vi "sv_Peak View Amplitude (Array).vi"(7 "peak units":enum16{"EU rms", "EU peak", "EU peak-peak"}(ring), 8 "error in (no error)":errorcluster, 9 "spectrum info":T1={"channel name"="", "description"="", "x-axis units"=0, "spectral info"={"spectrum type"=enum."Power [Magnitude^2]", "linear/dB"=enum."linear", "window"=0, "window size"=0, "FFT size"=0}, "engineering units"=0, "custom label"="", "dB reference [EU]"=0.0, "peak units"=enum."rms", "weighting filter"=0, "spectral density?"=FALSE, "unit label"="", "spectrum skewed?"=FALSE, "complimentary spectrum units"=enum."none"} {"x-axis units" items=["Time (s)"=0, "Frequency-CB (Hz)"=1, "Frequency-CPB (Hz)"=1248, "Frequency-Arbitrary (Hz)"=2357, "Quefrency (s)"=2, "Revolutions (rev)"=3, "Order"=4, "Speed (RPM)"=11, "Speed (rad/s)"=21, "Index"=65535]; "weighting filter" items=["Linear", "A-weighting", "B-weighting", "C-weighting", "ITU-R 468-4", "Dolby", "CCITT", "C-message", "Wb", "Wc", "Wd", "We", "Wf", "Wh", "Wj", "Wk", "Wm", "AES17 20 kHz lowpass", "AES17 40 kHz lowpass", "AES17 20 kHz highpass", "AES17 40 kHz highpass"]; "dB reference [EU]" format="%.2f"; "engineering units" items=["custom..."=0, "V"=1, "A"=21, "C"=30, "pC"=31, "s"=32, "-"=29, "Pa"=2, "N"=20, "g"=3, "m/s^2"=4, "m/s"=5, "m"=6, "mm/s"=12, "mm"=13, "micron/s"=14, "micron"=15, "in/s^2"=7, "in/s"=8, "in"=9, "mil/s"=10, "mil"=11, "rad/s^2"=16, "rad/s"=17, "rad"=18, "deg/s^2"=26, "deg/s"=27, "deg"=28, "RPM"=22, "cycle/s^2"=23, "Hz"=24, "cycle"=25, "strain"=19]; "spectral info"."window" items=["None "=0, "Hanning"=1, "Hamming"=2, "Blackman-Harris"=3, "Exact Blackman"=4, "Blackman"=5, "Flat Top"=6, "4 Term B-Harris "=7, "7 Term B-Harris"=8, "Low Sidelobe"=9, "Force - Exponential"=10, "Gaussian"=62]}, 11 "peak amplitudes [EU pk]":dbl[](array[numeric]) format="%.2f") -> (0 "error out":errorcluster, 3 "converted peak amplitudes":dbl[](array[numeric]) format="%.2f", 5 "unit label":string)   [LabVIEW 2017, in "SoundVib_Distortion.lvlib"]
uses:
  <vilib>/addons/Sound and Vibration/svt_Distortion/SoundVib_Distortion.lvlib
  <vilib>/addons/_NISVFA/_Shared subVIs/Controls/svc_Spectrum Info.ctl
  <vilib>/addons/_NISVFA/_Shared subVIs/Controls/svc_X-Axis Units.ctl
  <vilib>/addons/_NISVFA/_Shared subVIs/Controls/svc_Spectrum Type.ctl
  <vilib>/addons/_NISVFA/_Shared subVIs/Controls/svc_Engineering Units Text Ring.ctl
  <vilib>/addons/_NISVFA/_Shared subVIs/Controls/svc_Weighting Filter Text Ring.ctl
  <vilib>/addons/_NISVFA/_Shared subVIs/Controls/svc_Complimentary Spectrum Units.ctl
  <vilib>/addons/_NISVFA/_Shared subVIs/Common/svc_Get Weighting Enum and Labels.vi
  <vilib>/addons/_NISVFA/_Shared subVIs/Common/svc_Unit Label Lexical Class.vi
  <vilib>/addons/_NISVFA/_Shared subVIs/Common/svc_Engineering Units to Unit Label.vi
  <vilib>/addons/_NISVFA/_Shared subVIs/Common/svc_Format Value (DBL).vi
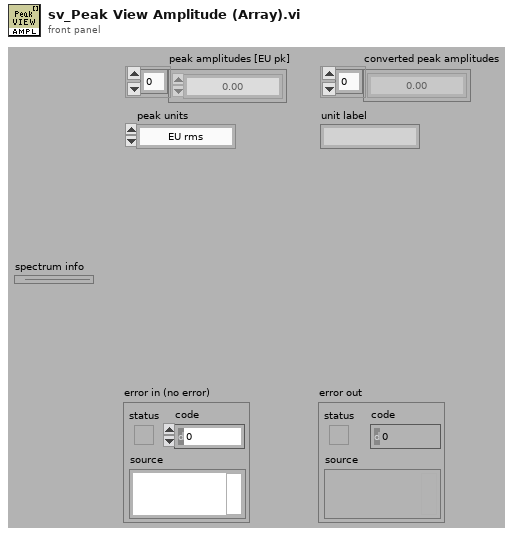
[diagram p1: front panel]
types:
  T1 = typedef "svc_Spectrum Info.ctl" = cluster{"channel name":string, "description":string, "x-axis units":T2, "spectral info":cluster{"spectrum type":T3, "linear/dB":enum16{"linear", "dB"}, "window":u16, "window size":i32, "FFT size":i32}, "engineering units":T4, "custom label":string, "dB reference [EU]":dbl, "peak units":enum16{"rms", "peak", "peak-peak"}, "weighting filter":T5, "spectral density?":bool, "unit label":string, "spectrum skewed?":bool, "complimentary spectrum units":T6}
  T2 = typedef "svc_X-Axis Units.ctl" = u16
  T3 = typedef "svc_Spectrum Type.ctl" = enum16{"FFT Spectrum [complex]", "Amplitude [Magnitude]", "Power [Magnitude^2]", "Cross Spectrum [complex]", "Frequency Response [Complex]"}
  T4 = typedef "svc_Engineering Units Text Ring.ctl" = u16
  T5 = typedef "svc_Weighting Filter Text Ring.ctl" = u16
  T6 = typedef "svc_Complimentary Spectrum Units.ctl" = enum16{"none", "radians", "degrees", "cycles", "imaginary"}
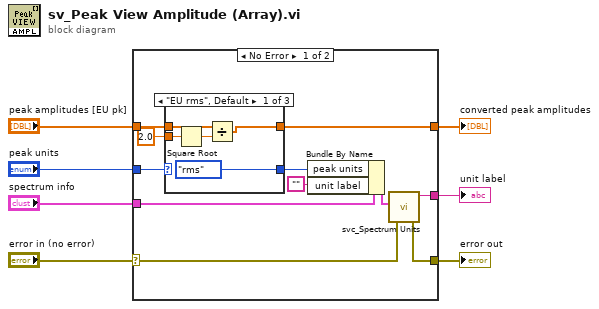
[diagram p0: block diagram]
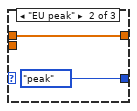
[diagram p2: hidden frame]
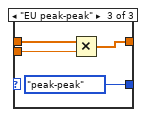
[diagram p3: hidden frame]
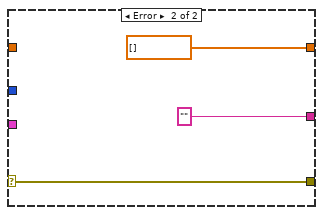
[diagram p4: hidden frame]
diagram:
  n1 = case shown="No Error" "error in (no error)" {
    selector: "error in (no error)" -> [w13 w30]
    tunnel: [w14 ""] -> w7
    tunnel: [w17 dbl[] [] ("peak amplitudes [EU pk]")] -> w1
    tunnel: "peak amplitudes [EU pk]" -> [w16 _]
    tunnel: "peak units" -> [w15 _]
    tunnel: [w12 w30] -> w4
    tunnel: "spectrum info" -> [w11 _]
    frame No Error {
      n2 = case shown="\"EU rms\", Default" w15 {
        tunnel: w16 -> [w23 w25 w28]
        tunnel: [w20 w25 w27] -> w17
        tunnel: 2.0 ("y") -> [w21 _ w29]
        tunnel: [enum16{"rms", "peak", "peak-peak"}."rms" ("peak units") enum16{"rms", "peak", "peak-peak"}."peak" ("peak units") enum16{"rms", "peak", "peak-peak"}."peak-peak" ("peak units")] -> w9
        frame "EU rms", Default {
          n3 = Square Root(x=w21) -> (sqrt(x)=w22:dbl)
          n4 = Divide(x=w23, y=w22) -> (x/y=w20:dbl[])
        }
        frame "EU peak" {
        }
        frame "EU peak-peak" {
          n5 = Multiply(x=w28, y=w29) -> (x*y=w27:dbl[])
        }
      }
      n6 = Bundle By Name(cluster=w11, "peak units"=w9, "unit label"="") -> (w10:T1)
      n7 = call <vilib>:"svc_Spectrum Units.vi"("error in (no error)"=w13, "spectrum info in"=w10) -> ("error out"=w12:errorcluster, "unit label"=w14:string)  [unwired: 2 in, 2 out]
    }
    frame Error {
    }
  }
  "unit label" <- w7
  "error out" <- w4
  "converted peak amplitudes" <- w1
